vi "Connect.vi"(10 "error in (no error)":errorcluster, 11 "WAMP Client in":refnum<class "WAMP Client.lvclass">) -> (2 "error out":errorcluster, 3 "WAMP Client out":refnum<class "WAMP Client.lvclass">)   [LabVIEW 2020, in "WAMP Client.lvclass"]
doc: "Connects to the WAMP router and performs the HELLO/WELCOME handshake. After calling this the WAMP session is ready for use."
uses:
  <userlib>/lvwamp/WAMP Client/WAMP Client.lvclass
  <userlib>/lvwamp/WAMP Client/WAMP Client.lvclass/WAMP Client.ctl
  <userlib>/lvwamp/WAMP Client/TypeDef/ABORT Request Data.ctl
  <userlib>/lvwamp/Comm Handlers/ICommHandler/ICommHandler.lvclass
panel:
  in  "Boolean":bool
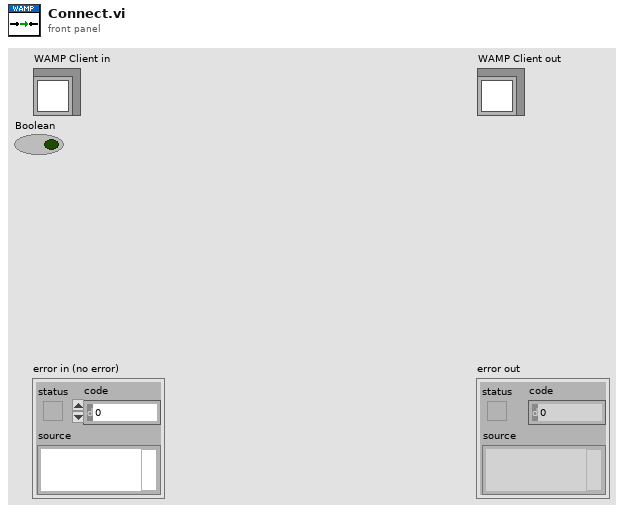
[diagram p1: front panel]
types:
  T1 = typedef "WAMP Client.lvclass/ABORT Request Data.ctl" = cluster{"Error URI":string, "Message":string}
  T2 = typedef "WAMP Client.lvclass/WAMP Received Message.ctl" = cluster{"Message JSON":string[], "Message Codes":T3}
  T3 = typedef "WAMP Client.lvclass/WAMP Message Codes.ctl" = u16
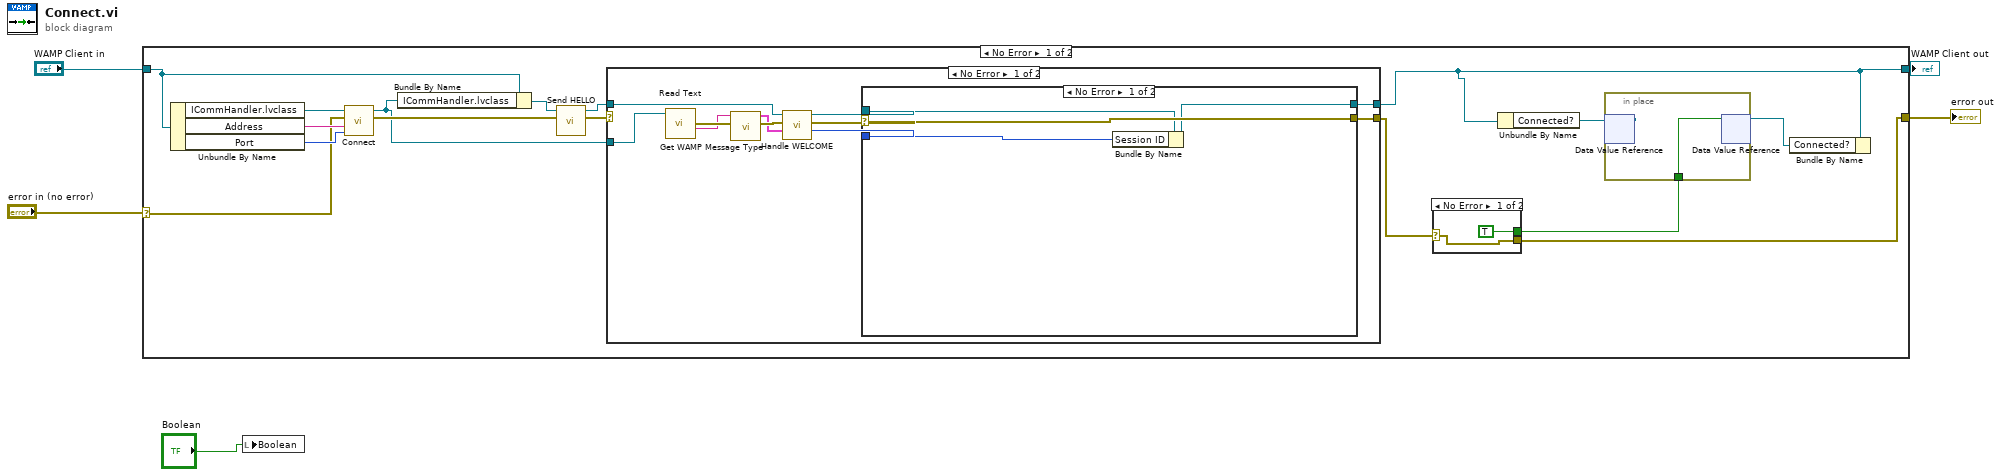
[diagram p0: block diagram]
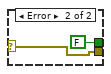
[diagram p2: hidden frame]
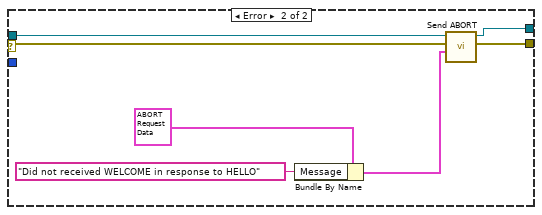
[diagram p3: hidden frame]
diagram:
  n1 = case shown="No Error" "error in (no error)" {
    selector: "error in (no error)" -> [w12 w52]
    tunnel: [w9 w52] -> w4
    tunnel: [w10 w51] -> w2
    tunnel: "WAMP Client in" -> [w16 w51]
    frame No Error {
      n2 = Unbundle By Name(w16) -> ("ICommHandler.lvclass"=w19:refnum<class "ICommHandler.lvclass">, "Address"=w18:string, "Port"=w17:u16)
      n3 = call-dynamic "Connect.vi"("Port"=w17, "Address"=w18, "error in"=w12, "ICommHandler in"=w19) -> ("error out"=w15:errorcluster, "ICommHandler out"=w13:refnum<class "ICommHandler.lvclass">)  [unwired: 4 in]
      n4 = Bundle By Name(cluster=w16, "ICommHandler.lvclass"=w13) -> (w14:refnum<class "WAMP Client.lvclass">)
      n5 = call-dynamic "Send HELLO.vi"("error in (no error)"=w15, "WAMP Client in"=w14) -> ("error out"=w21:errorcluster, "WAMP Client out"=w20:refnum<class "WAMP Client.lvclass">)  [unwired: 8 in]
      n6 = case shown="No Error" w21 {
        selector: w21 -> [_ w49]
        tunnel: w20 -> [w33 w50]
        tunnel: [w29 w50] -> w10
        tunnel: [w31 w49] -> w11
        tunnel: w13 -> [w37 _]
        frame No Error {
          n7 = call-dynamic "Read Text.vi"("ICommHandler in"=w37) -> ("String"=w35:string, "error out"=w36:errorcluster)  [unwired: 6 in, 1 out]
          n8 = call <userlib>:"Get WAMP Message Type.vi"("error in (no error)"=w36, "JSON"=w35) -> ("error out"=w34:errorcluster, "WAMP Message"=w27:T2)  [unwired: 6 in, 2 out]
          n9 = call-dynamic "Handle WELCOME.vi"("WAMP Message"=w27, "error in (no error)"=w34, "WAMP Client in"=w33) -> ("Session ID"=w28:u32, "error out"=w32:errorcluster, "WAMP Client out"=w30:refnum<class "WAMP Client.lvclass">)  [unwired: 6 in]
          n10 = case shown="No Error" w32 {
            selector: w32 -> [w41 w44]
            tunnel: [w41 w46] -> w31
            tunnel: w30 -> [w38 w45]
            tunnel: [w40 w43] -> w29
            tunnel: w28 -> [w39 _]
            frame No Error {
              n11 = Bundle By Name(cluster=w38, "Session ID"=w39) -> (w40:refnum<class "WAMP Client.lvclass">)
            }
            frame Error {
              n12 = Bundle By Name(cluster=T1 {"Error URI"="wamp.error.protocol_violation", "Message"=""} ("Cluster"), "Message"="Did not received WELCOME in response to HELLO") -> (w42:T1)
              n13 = call-dynamic "Send ABORT.vi"("Abort Request"=w42, "error in (no error)"=w44, "WAMP Client in"=w45) -> ("error out"=w46:errorcluster, "WAMP Client out"=w43:refnum<class "WAMP Client.lvclass">)  [unwired: 7 in]
            }
          }
        }
        frame Error {
        }
      }
      n14 = case shown="No Error" w11 {
        selector: w11 -> [w23 w25]
        tunnel: [TRUE FALSE] -> w6
        tunnel: [w23 w25] -> w9
        frame No Error {
        }
        frame Error {
        }
      }
      n15 = Unbundle By Name(w10) -> ("Connected?"=w8:refnum<data-value>)
      n16 = in-place {
        in-place-border: w6 -> [w22]
        n17 = in-place-dvr #1(w8) -> ()  [unwired: 2 out]
        n18 = in-place-dvr #1(w22) -> (w7:refnum<data-value>)  [unwired: 1 out]
      }
      n19 = Bundle By Name(cluster=w10, "Connected?"=w7) -> ()  [unwired: 1 out]
    }
    frame Error {
    }
  }
  "error out" <- w4
  "WAMP Client out" <- w2
  n20 = local write "Boolean"("Boolean") -> ()
